vi "Open Default ColorProcessors.vi"(6 "Bit Depth":i32, 8 "error in (no error)":errorcluster, 9 "Color Correction Matrix":sgl[](array[numeric]), 10 "White Balance Matrix":sgl[](array[numeric]), 11 "ColorProcessorSDK reference":refnum<k24>) -> (0 "error out":errorcluster, 1 "LinearRGBColorProcessor":refnum<k24>, 2 "StandardRGBColorProcessor":refnum<k24>, 3 "ColorProcessorSDK reference out":refnum<k24>)   [LabVIEW 2022 SP3]
uses:
  I:/.shortcut-targets-by-id/1riZacJd_1_jmKfGgrjDuP7KcecvMS3i2/Xiao research group/Programs/XYZRecorrection/Scientific Camera Interfaces/SDK/DotNet Toolkit/dlls/Managed_64_lib/Thorlabs.TSI.ColorProcessor.dll
  SDK/DotNet Toolkit/dlls/Managed_64_lib/Thorlabs.TSI.ColorProcessor.dll
  I:/.shortcut-targets-by-id/1riZacJd_1_jmKfGgrjDuP7KcecvMS3i2/Xiao research group/Programs/XYZRecorrection/Scientific Camera Interfaces/SDK/DotNet Toolkit/dlls/Managed_64_lib/Thorlabs.TSI.ColorInterfaces.dll
  SDK/DotNet Toolkit/dlls/Managed_64_lib/Thorlabs.TSI.ColorInterfaces.dll
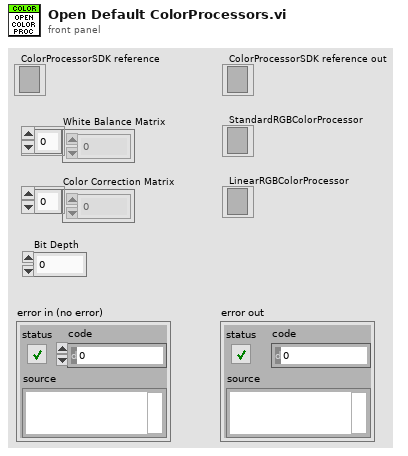
[diagram p1: front panel]
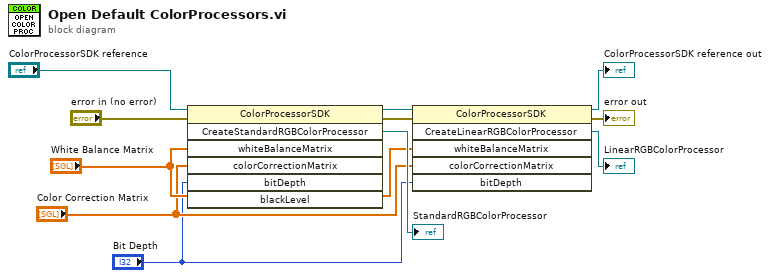
[diagram p0: block diagram]
diagram:
  n1 = invoke class="ColorProcessorSDK" method="CreateStandardRGBColorProcessor"(reference="ColorProcessorSDK reference", error in="error in (no error)", "whiteBalanceMatrix"="White Balance Matrix", "colorCorrectionMatrix"="Color Correction Matrix", "bitDepth"="Bit Depth") -> (reference out=w9:refnum<k24>, error out=w8:errorcluster, "CreateStandardRGBColorProcessor"=→"StandardRGBColorProcessor":refnum<k24>)  [unwired: 2 in, 4 out]
  n2 = invoke class="ColorProcessorSDK" method="CreateLinearRGBColorProcessor"(reference=w9, error in=w8, "whiteBalanceMatrix"="White Balance Matrix", "colorCorrectionMatrix"="Color Correction Matrix", "bitDepth"="Bit Depth") -> (reference out=→"ColorProcessorSDK reference out":refnum<k24>, error out=→"error out":errorcluster, "CreateLinearRGBColorProcessor"=→"LinearRGBColorProcessor":refnum<k24>)  [unwired: 1 in, 3 out]
